vi "IOScan_usToMoreAppropriateUnits.vi"(10 "Period (us)":u32) -> (2 "Units":T1 items=["us", "ms", "secs"], 3 "Period":u32)   [LabVIEW 2016]
uses:
  <resource>/dialog/TargetPreferencePages/IOScan_SubVIs/IOScan_TimeUnit.ctl
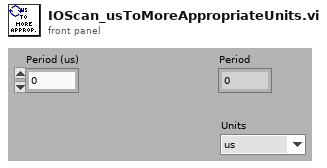
[diagram p1: front panel]
types:
  T1 = typedef "IOScan_TimeUnit.ctl" = u16
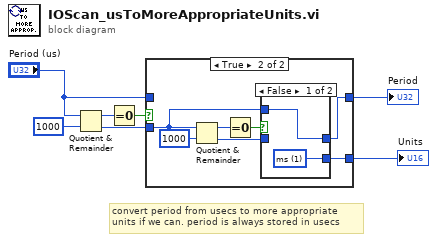
[diagram p0: block diagram]
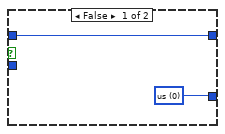
[diagram p2: hidden frame]
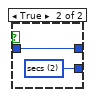
[diagram p3: hidden frame]
diagram:
  # "convert period from usecs to more appropriate units if we can. period is always stored in usecs"
  n1 = Quotient & Remainder(x="Period (us)", y=u32 1000) -> (x-y*floor(x/y)=w6:u32, floor(x/y)=w4:u32)
  n2 = Equal To 0?(x=w6) -> (x = 0?=w5:bool)
  n3 = case shown="True" w5 {
    tunnel: w4 -> [_ w10]
    tunnel: [w9 w12] -> w3
    tunnel: [w8 w11] -> w2
    tunnel: "Period (us)" -> [w9 _]
    frame False {
      w8 = T1 0 items=["us", "ms", "secs"] ("Units")
    }
    frame True {
      n4 = Quotient & Remainder(x=w10, y=u32 1000) -> (x-y*floor(x/y)=w16:u32, floor(x/y)=w13:u32)
      n5 = Equal To 0?(x=w16) -> (x = 0?=w14:bool)
      n6 = case shown="False" w14 {
        tunnel: w13 -> [_ w20]
        tunnel: [w18 w20] -> w12
        tunnel: [w17 w19] -> w11
        tunnel: w10 -> [w18 _]
        frame False {
          w17 = T1 1 items=["us", "ms", "secs"] ("Units")
        }
        frame True {
          w19 = T1 2 items=["us", "ms", "secs"] ("Units")
        }
      }
    }
  }
  "Period" <- w3
  "Units" <- w2
